vi "TCP Named Service - Client.vi"() -> ()   [LabVIEW 2013]
doc: "本VI可用于实现TCP Named Service - Server.vi的一个客户端。该客户端可通过服务器地址和服务名称连接该服务。客户端接收服务器发送的字符串、显示字符串并关闭连接。"
panel:
  out "服务器消息":string
  # "概述：演示使用TCP函数通过命名服务连接至TCP服务器VI并接收数据。\n操作步骤：\n1. 确保已运行TCP Named Service - Server.vi。\n2. 运行VI。"
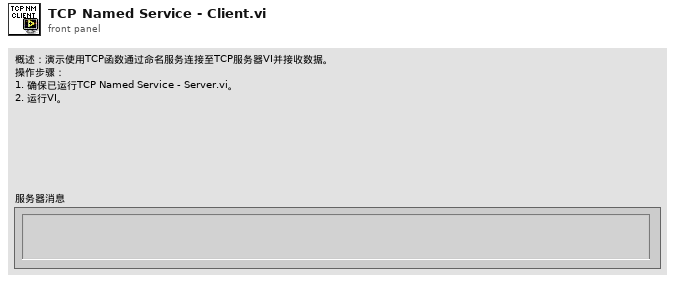
[diagram p1: front panel]
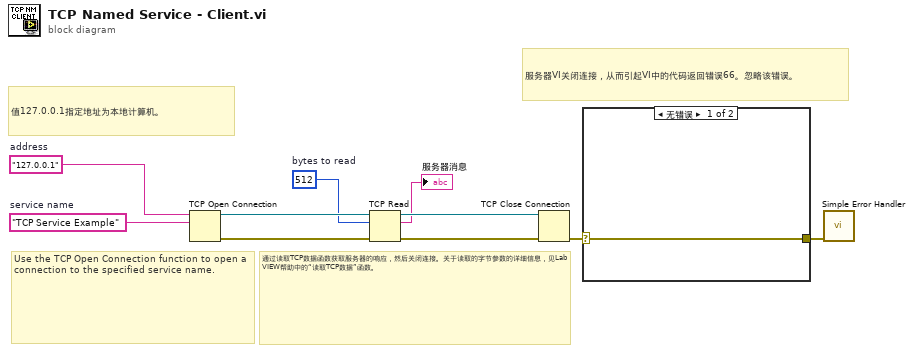
[diagram p0: block diagram]
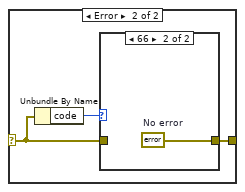
[diagram p2: hidden frame]
diagram:
  w3 = 512  # bytes to read
  w4 = "TCP Service Example"  # service name
  w5 = "127.0.0.1"  # address
  # "服务器VI关闭连接，从而引起VI中的代码返回错误66。忽略该错误。"
  # "值127.0.0.1指定地址为本地计算机。"
  # "Use the TCP Open Connection function to open a connection to the specified service name."
  # "通过读取TCP数据函数获取服务器的响应，然后关闭连接。关于读取的字节参数的详细信息，见LabVIEW帮助中的“读取TCP数据”函数。"
  n1 = TCP Open Connection(address=w5, remote port or service name=w4) -> (connection ID=w9:refnum<k5>, error out=w10:errorcluster)  [unwired: 3 in]
  n2 = TCP Read(connection ID=w9, bytes to read=w3, error in (no error)=w10) -> (connection ID out=w8:refnum<k5>, data out=→"服务器消息":string, error out=w7:errorcluster)  [unwired: 2 in]
  n3 = TCP Close Connection(connection ID=w8, error in (no error)=w7) -> (error out=w2:errorcluster)  [unwired: 1 in, 1 out]
  n4 = case shown="无错误" w2 {
    selector: w2 -> [w11 w13]
    tunnel: [w11 w12] -> w1
    frame No Error {
    }
    frame Error {
      n5 = Unbundle By Name(w13) -> ("code"=w14:i32)
      n6 = case shown="66" w14 {
        tunnel: w13 -> [w15 _]
        tunnel: [w15 w16] -> w12
        frame Default {
        }
        frame 66 {
          w16 = errorcluster {"status"=FALSE, "code"=0, "source"=""}  # No error
        }
      }
    }
  }
  n7 = call <vilib>:"Simple Error Handler.vi"("error in (no error)"=w1) -> ()  [unwired: 4 in, 5 out]
